vi "Line Follow.vi"(8 "error in":errorcluster, 9 "Speed":dbl, 10 "Move":T1(ring), 11 "FPGA VI Reference Out 2":refnum<k20>) -> (0 "error out":errorcluster, 3 "FPGA VI Reference Out":refnum<k20>)   [LabVIEW 2019]
uses:
  <vilib>/Platform/TimedLoop/XDataNode/timing_clust.ctl
  <vilib>/Platform/TimedLoop/XDataNode/nitl_modes.ctl
  <vilib>/Platform/TimedLoop/XDataNode/wakeup.ctl
  <vilib>/robotics/Steering/Mecanum Wheel/Roller Orientation.ctl
  <vilib>/robotics/Steering/Wheel/Wheel Parameters.ctl
  <vilib>/robotics/Steering/Wheel/Rotation Direction.ctl
  <vilib>/robotics/Steering/Mecanum Steering Frame/NI_Robotics_Mecanum Steering Frame.lvclass
  C:/Program Files (x86)/National Instruments/LabVIEW 2019/vi.lib/robotics/Steering/Steering Frame/NI_Robotics_Steering Frame.lvclass
  <vilib>/robotics/Steering/Mecanum Wheel/Create Mecanum Wheel.vi
  <vilib>/robotics/Steering/Mecanum Steering Frame/Create Mecanum Steering Frame.vi
  <vilib>/Utility/error.llb/Error Cluster From Error Code.vi
  <vilib>/rvi/errors/niLvFpgaAdjustHostInterfaceError.vi
  <vilib>/robotics/Steering/Steering Frame/Apply Steering Frame Velocity to Motors.vi
  <vilib>/platform/TimedLoop/XDataNode/XDataNode.xnode
  <vilib>/robotics/Steering/Create Steering Frame/NI_Robotics_Create Steering Frame.xnode
  <vilib>/robotics/Steering/Class Type Definitions/Mecanum Steering Frame.ctl
  <vilib>/rvi/interface/nirviReadWriteControl/nirviReadWriteControl.xnode
  <vilib>/Platform/TimedLoop/XDataNode/XDNodeRunTimeDep.lvlib
  <vilib>/robotics/Steering/Steering Frame/NI_Robotics_Steering Frame.lvclass
  NiFpgaLv.dll
  <vilib>/rvi/interface/Simulation/niFpgaSimulationCallBeginRW.vi
  <vilib>/robotics/Steering/Class Type Definitions/NI_Robotics_Steering Class Types.lvlib
  <vilib>/robotics/Steering/Mecanum Wheel/NI_Robotics_Mecanum Wheel.lvclass
  <vilib>/robotics/Steering/Wheel/NI_Robotics_Wheel.lvclass
  C:/Program Files (x86)/National Instruments/LabVIEW 2019/vi.lib/robotics/Steering/Special Steering Frame/NI_Robotics_Special Steering Frame.lvclass
panel:
  in  "Stop":bool
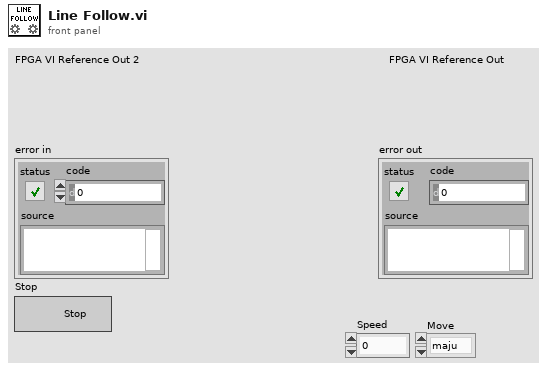
[diagram p1: front panel]
types:
  T1 = enum16{"maju", "mundur", "kanan", "kiri", "atas kanan", "atas kiri", "bawah kanan", "bawah kiri", "putar kanan", "putar kiri"}
  T2 = typedef "NI_Robotics_Steering Class Types.lvlib/Mecanum Steering Frame.ctl" = refnum<class "NI_Robotics_Mecanum Steering Frame.lvclass">
  T3 = typedef "XDNodeRunTimeDep.lvlib/timing_clust.ctl" = cluster{"Expected End [f-1]":u64, "Actual End [f-1]":u64, "Finished Late? [f-1]":bool, "Expected End [i-1]":u64, "Actual End [i-1]":u64, "Finished Late? [i-1]":bool, "Expected Start [i]":u64, "Actual Start [i]":u64, "Expected Start [f]":u64, "Actual Start [f]":u64, "Source Name":string, "Structure Name":string, "Period":i64, "Deadline":i64, "Offset":i64, "Start":i64, "Priority":i32, "Timeout":i32, "Mode":T4, "Wakeup Reason":T5, "Error":errorcluster, "Source Type":string, "Secondary Source Type":string, "Global End Time":u64, "Global Start Time":u64, "Frame Duration":u64, "Iteration Duration":u64, "Assigned CPU":i32, "I/O Scan Engine Mode":u32}
  T4 = typedef "XDNodeRunTimeDep.lvlib/nitl_modes.ctl" = enum32{"No Change", "Process missed periods, maintain original phase", "Discard missed periods, maintain original phase", "Process missed periods, ignore original phase", "Discard missed periods, ignore original phase"}
  T5 = typedef "XDNodeRunTimeDep.lvlib/wakeup.ctl" = enum32{"Normal", "Aborted", "Asynchronous wakeup", "Timing source error", "Timed loop error", "Timeout"}
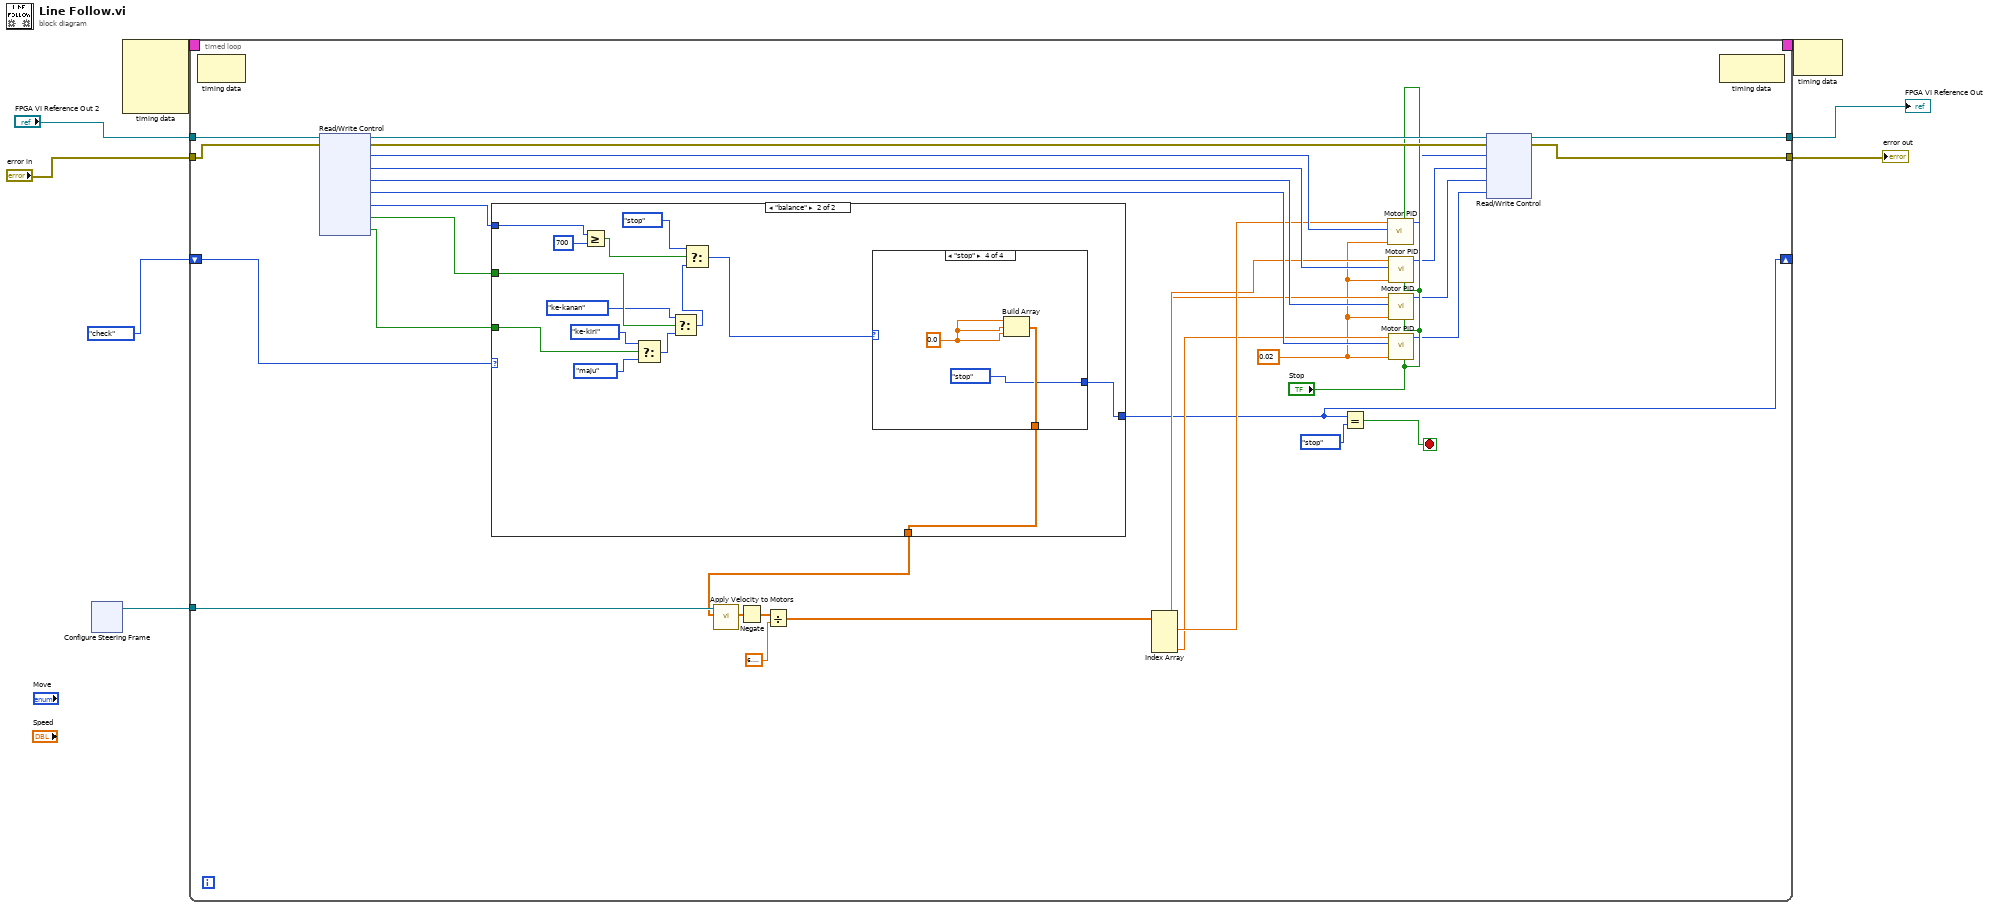
[diagram p0: block diagram]
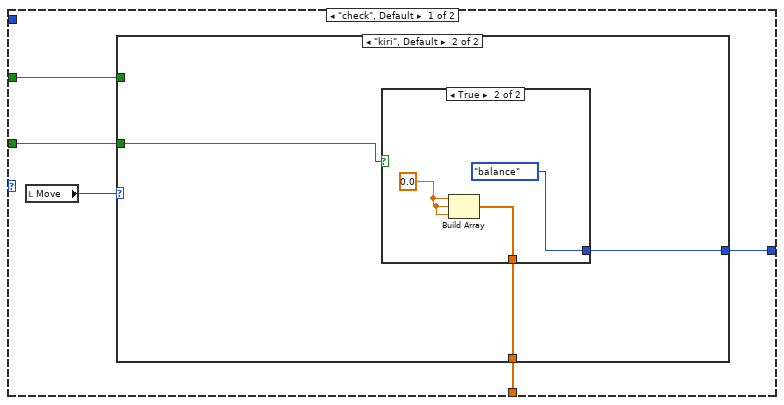
[diagram p2: hidden frame]
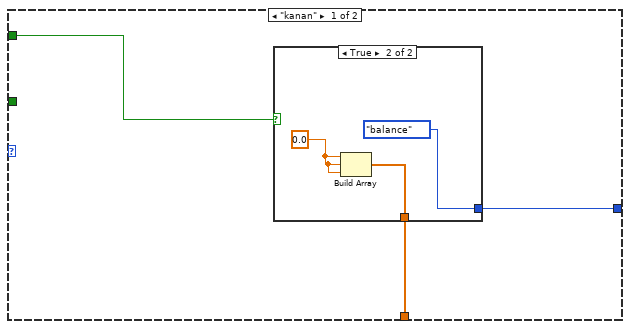
[diagram p3: hidden frame]
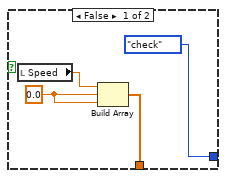
[diagram p4: hidden frame]
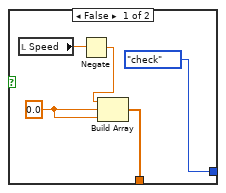
[diagram p5: hidden frame]
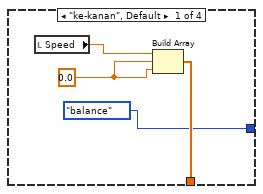
[diagram p6: hidden frame]
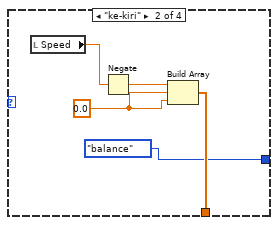
[diagram p7: hidden frame]
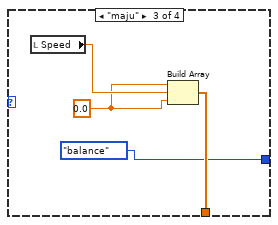
[diagram p8: hidden frame]
diagram:
  n1 = xnode ("Configure Steering Frame")() -> ("mecanum steering frame out"=w6:T2)  [unwired: 1 in, 1 out]
  n2 = node-c288() -> (w8:T3)  [unwired: 4 in]
  n3 = timed-loop {
    timing: w8 -> [_]
    timing-out: [_] -> w7
    tunnel: w6 -> [w41]
    tunnel: "FPGA VI Reference Out 2" -> [w38]
    tunnel: [w40] -> w5
    tunnel: "error in" -> [w37]
    tunnel: [w39] -> w4
    shift-right: [w13] -> _
    shift-left: enum16{"check", "balance", "stop"}."check" -> [w16]
    stop <- w9 stop-if-true
    w17 = 0.02 ("dt[s]")
    n4 = node-c288() -> ()  [unwired: 1 in, 1 out]
    n5 = xnode "Read/Write Control"("FPGA VI Reference In"=w38, "error in"=w37) -> ("FPGA VI Reference Out"=w35:refnum<k20>, "error out"=w34:errorcluster, "ENC M1"=w33:i32, "ENC M2"=w32:i32, "ENC M3"=w31:i32, "ENC M4"=w30:i32, "IR 1"=w10:u16, "LINE 1"=w15:bool, "LINE 2"=w11:bool)
    n6 = case shown="\"balance\"" w16 {
      tunnel: w15 -> [w45 w78]
      tunnel: [w44 w68] -> w13
      tunnel: [w43 w69] -> w12
      tunnel: w11 -> [w42 w80]
      tunnel: w10 -> [_ w74]
      frame "check", Default {
        n7 = local read "Move"() -> (w46:T1)
        n8 = case shown="\"kiri\", Default" w46 {
          tunnel: w45 -> [w49 _]
          tunnel: [w48 w59] -> w44
          tunnel: [w47 w58] -> w43
          tunnel: w42 -> [_ w57]
          frame "kanan" {
            n9 = case shown="True" w49 {
              tunnel: [enum16{"check", "balance", "stop"}."check" enum16{"check", "balance", "stop"}."balance"] -> w48
              tunnel: [w50 w54] -> w47
              frame False {
                w51 = 0.0 ("element")
                n10 = local read "Speed"() -> (w52:dbl)
                n11 = Build Array(w52, w51, w51) -> (w50:dbl[])
              }
              frame True {
                w55 = 0.0 ("element")
                n12 = Build Array(w55, w55, w55) -> (w54:dbl[])
              }
            }
          }
          frame "kiri", Default {
            n13 = case shown="True" w57 {
              tunnel: [enum16{"check", "balance", "stop"}."check" enum16{"check", "balance", "stop"}."balance"] -> w59
              tunnel: [w61 w65] -> w58
              frame False {
                w62 = 0.0 ("element")
                n14 = local read "Speed"() -> (w63:dbl)
                n15 = Negate(x=w63) -> (-x=w60:dbl)
                n16 = Build Array(w60, w62, w62) -> (w61:dbl[])
              }
              frame True {
                w66 = 0.0 ("element")
                n17 = Build Array(w66, w66, w66) -> (w65:dbl[])
              }
            }
          }
        }
      }
      frame "balance" {
        n18 = Greater Or Equal?(x=w74, y=u16 700) -> (x >= y?=w72:bool)
        n19 = Select(t=enum16{"ke-kanan", "ke-kiri", "maju", "stop"}."ke-kiri", s=w80, f=enum16{"ke-kanan", "ke-kiri", "maju", "stop"}."maju") -> (s? t:f=w77:enum16{"ke-kanan", "ke-kiri", "maju", "stop"})
        n20 = Select(t=enum16{"ke-kanan", "ke-kiri", "maju", "stop"}."ke-kanan", s=w78, f=w77) -> (s? t:f=w71:enum16{"ke-kanan", "ke-kiri", "maju", "stop"})
        n21 = Select(t=enum16{"ke-kanan", "ke-kiri", "maju", "stop"}."stop", s=w72, f=w71) -> (s? t:f=w70:enum16{"ke-kanan", "ke-kiri", "maju", "stop"})
        n22 = case shown="\"stop\"" w70 {
          tunnel: [w83 w88 w94 w97] -> w69
          tunnel: [enum16{"check", "balance", "stop"}."balance" enum16{"check", "balance", "stop"}."balance" enum16{"check", "balance", "stop"}."balance" enum16{"check", "balance", "stop"}."stop"] -> w68
          frame "ke-kanan", Default {
            w84 = 0.0 ("element")
            n23 = local read "Speed"() -> (w85:dbl)
            n24 = Build Array(w85, w84, w84) -> (w83:dbl[])
          }
          frame "ke-kiri" {
            w89 = 0.0 ("element")
            n25 = local read "Speed"() -> (w90:dbl)
            n26 = Negate(x=w90) -> (-x=w87:dbl)
            n27 = Build Array(w87, w89, w89) -> (w88:dbl[])
          }
          frame "maju" {
            w92 = 0.0 ("element")
            n28 = local read "Speed"() -> (w93:dbl)
            n29 = Build Array(w92, w93, w92) -> (w94:dbl[])
          }
          frame "stop" {
            w96 = 0.0 ("element")
            n30 = Build Array(w96, w96, w96) -> (w97:dbl[])
          }
        }
      }
    }
    n31 = call-poly <vilib>:"Apply Velocity to Motors.vi"("steering frame velocity"=w12, "steering frame in"=w41) -> ("ccw motor velocity setpoints"=w36:dbl[])  [unwired: 5 in, 4 out]
    n32 = Negate(x=w36) -> (-x=w29:dbl[])
    n33 = Divide(x=w29, y=6.283185307179586) -> (x/y=w27:dbl[])
    n34 = Index Array(array=w27) -> (element #1=w26:dbl, element #2=w25:dbl, element #3=w24:dbl, element #4=w23:dbl)  [unwired: 4 in]
    n35 = Equal?(x=w13, y=enum16{"check", "balance", "stop"}."stop") -> (x = y?=w9:bool)
    n36 = call "Motor PID.vi"("Stop"="Stop", "dt[s]"=w17, "encoder"=w33, "vel ref[rps]"=w26) -> ("duty cycle"=w21:i16)  [unwired: 5 in, 2 out]
    n37 = call "Motor PID.vi"("Stop"="Stop", "dt[s]"=w17, "encoder"=w32, "vel ref[rps]"=w25) -> ("duty cycle"=w20:i16)  [unwired: 5 in, 2 out]
    n38 = call "Motor PID.vi"("Stop"="Stop", "dt[s]"=w17, "encoder"=w31, "vel ref[rps]"=w24) -> ("duty cycle"=w19:i16)  [unwired: 5 in, 2 out]
    n39 = call "Motor PID.vi"("Stop"="Stop", "dt[s]"=w17, "encoder"=w30, "vel ref[rps]"=w23) -> ("duty cycle"=w18:i16)  [unwired: 5 in, 2 out]
    n40 = xnode "Read/Write Control"("FPGA VI Reference In"=w35, "error in"=w34, "M1"=w21, "M2"=w20, "M3"=w19, "M4"=w18) -> ("FPGA VI Reference Out"=w40:refnum<k20>, "error out"=w39:errorcluster)
    n41 = node-c288() -> ()  [unwired: 1 in, 1 out]
  }
  "error out" <- w4
  "FPGA VI Reference Out" <- w5
  n42 = node-c288(w7) -> ()  [unwired: 1 out]
